vi "tm3samp_sequence_wDSP.vi"() -> ()   [LabVIEW 2011]
panel:
  in  "SC Enable":bool
  in  "BG Enable":bool
  in  "Frame Averaging":i32(ring)=1 items=["1 Frame"=1, "2 Frames"=2, "4 Frames"=4]
  in  "Recursive Frames":i32(ring)=1 items=["1 Frame"=1, "2 Frames"=2, "4 Frames"=4, "8 Frames"=8, "16 Frames"=16]
  out "Image":u16[][](graph)
  in  "Quit":bool
  out "Error Out":errorcluster {"code" format="%.0x"}
  # "This is an example how to use the DSP functions.\nNot all camera have the DSP functions. Please\ncheck your camera manual to see your camera's\ncapabilities."
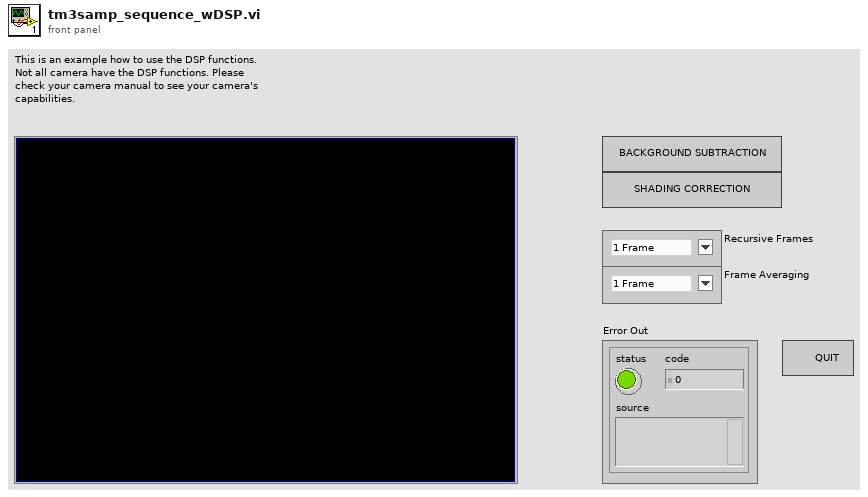
[diagram p1: front panel]
types:
  T1 = cluster{"width":u32, "height":u32, "datatype":u32}
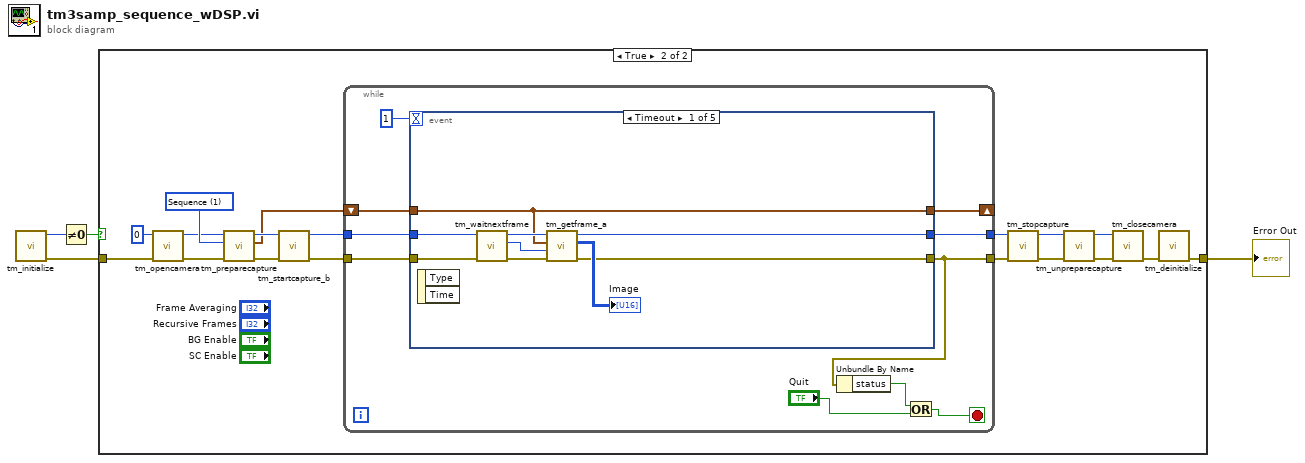
[diagram p0: block diagram]
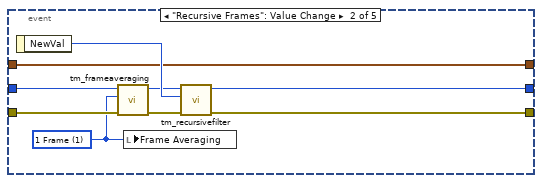
[diagram p3: hidden frame]
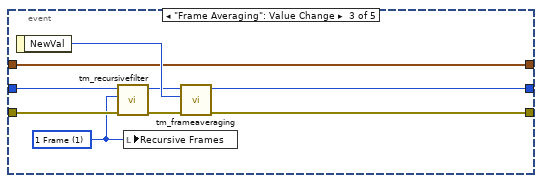
[diagram p4: hidden frame]
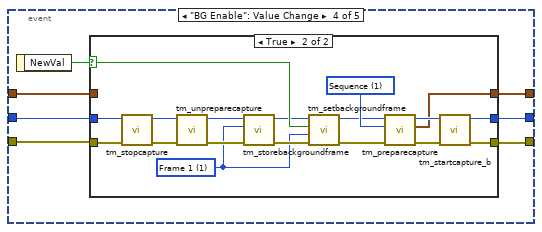
[diagram p5: hidden frame]
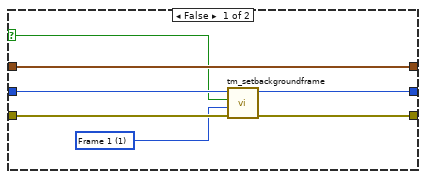
[diagram p6: hidden frame]
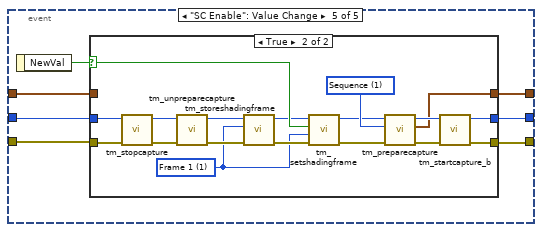
[diagram p7: hidden frame]
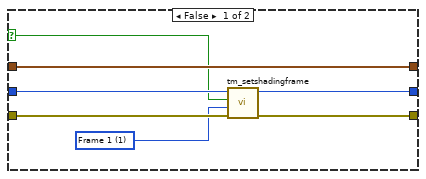
[diagram p8: hidden frame]
diagram:
  n1 = call <userlib>:"tm_initialize.vi"() -> ("error out"=w1:errorcluster, "Number Of Cameras"=w2:u32)  [unwired: 10 in]
  n2 = Not Equal To 0?(x=w2) -> (x != 0?=w4:bool)
  n3 = case shown="True" w4 {
    tunnel: w1 -> [w5 w23]
    tunnel: [w5 w20] -> w3
    frame False {
    }
    frame True {
      w13 = 1 items=["Snap", "Sequence"] ("Capture mode")
      n4 = call <userlib>:"tm_opencamera.vi"("error in (no error)"=w23, "Camera Index"=u32 0) -> ("error out"=w10:errorcluster, "Handle out"=w9:u32)  [unwired: 8 in]
      n5 = call <userlib>:"tm_preparecapture.vi"("error in (no error)"=w10, "Capture mode"=w13, "Handle in"=w9) -> ("error out"=w11:errorcluster, "Buffer"=w6:T1, "Handle out"=w12:u32)  [unwired: 5 in, 1 out]
      n6 = call <userlib>:"tm_startcapture_b.vi"("error in (no error)"=w11, "Handle in"=w12) -> ("error out"=w7:errorcluster, "Handle out"=w8:u32)  [unwired: 8 in]
      n7 = while {
        tunnel: [w31] -> w16
        tunnel: [w26] -> w17
        tunnel: w8 -> [w33]
        tunnel: w7 -> [w32]
        shift-right: [w25] -> _
        shift-left: w6 -> [w30]
        stop <- w24 stop-if-true
        n8 = event shown="[0] Timeout" {
          selector: _ -> [_ _ _ _ _]
          dyn-events: _ -> [_ _ _ _ _]
          timeout: 1 -> [_ _ _ _ _]
          tunnel: w33 -> [w38 w47 w56 w65 w97]
          tunnel: w32 -> [w37 w48 w57 w64 w96]
          tunnel: [w35 w50 w59 w62 w94] -> w31
          tunnel: [w36 w49 w58 w61 w93] -> w26
          tunnel: w30 -> [w34 w43 w52 w66 w98]
          tunnel: [w34 w43 w52 w63 w95] -> w25
          event Timeout {
            n9 = event-data() -> ()  [unwired: 1 in, 2 out]
            n10 = call <userlib>:"tm_waitnextframe.vi"("error in (no error)"=w37, "Handle in"=w38) -> ("error out"=w40:errorcluster, "Frame Index"=w42:i32, "Handle out"=w39:u32)  [unwired: 6 in, 1 out]
            n11 = call <userlib>:"tm_getframe_a.vi"("error in (no error)"=w40, "Frame Index"=w42, "Buffer"=w34, "Handle in"=w39) -> ("error out"=w36:errorcluster, "Data 16"=→"Image":u16[][], "Handle out"=w35:u32)  [unwired: 3 in, 2 out]
          }
          event "Recursive Frames": Value Change {
            w44 = 1 items=["1 Frame"=1, "2 Frames"=2, "4 Frames"=4, "8 Frames"=8, "16 Frames"=16] ("Frames")
            n12 = event-data() -> ("NewVal"=w51:i32)  [unwired: 1 in]
            n13 = call <userlib>:"tm_frameaveraging.vi"("error in (no error)"=w48, "Frames"=w44, "Handle in"=w47) -> ("error out"=w45:errorcluster, "Handle out"=w46:u32)  [unwired: 7 in]
            n14 = local write "Frame Averaging"(w44) -> ()
            n15 = call <userlib>:"tm_recursivefilter.vi"("error in (no error)"=w45, "Frames"=w51, "Handle in"=w46) -> ("error out"=w49:errorcluster, "Handle out"=w50:u32)  [unwired: 7 in]
          }
          event "Frame Averaging": Value Change {
            w53 = 1 items=["1 Frame"=1, "2 Frames"=2, "4 Frames"=4, "8 Frames"=8, "16 Frames"=16] ("Frames")
            n16 = event-data() -> ("NewVal"=w60:i32)  [unwired: 1 in]
            n17 = call <userlib>:"tm_recursivefilter.vi"("error in (no error)"=w57, "Frames"=w53, "Handle in"=w56) -> ("error out"=w54:errorcluster, "Handle out"=w55:u32)  [unwired: 7 in]
            n18 = local write "Recursive Frames"(w53) -> ()
            n19 = call <userlib>:"tm_frameaveraging.vi"("error in (no error)"=w54, "Frames"=w60, "Handle in"=w55) -> ("error out"=w58:errorcluster, "Handle out"=w59:u32)  [unwired: 7 in]
          }
          event "BG Enable": Value Change {
            n20 = event-data() -> ("NewVal"=w67:bool)  [unwired: 1 in]
            n21 = case shown="True" w67 {
              selector: w67 -> [w68 w86]
              tunnel: w65 -> [w74 w89]
              tunnel: w64 -> [w73 w90]
              tunnel: [w72 w77] -> w62
              tunnel: [w71 w76] -> w61
              tunnel: w66 -> [w70 _]
              tunnel: [w70 w75] -> w63
              frame False {
                w69 = 1 items=["Frame 1"=1, "Frame 2"=2, "Frame 3"=3, "Frame 4"=4] ("Frame")
                n22 = call <userlib>:"tm_setbackgroundframe.vi"("error in (no error)"=w73, "Frame"=w69, "Enable"=w68, "Handle in"=w74) -> ("error out"=w71:errorcluster, "Handle out"=w72:u32)  [unwired: 6 in]
              }
              frame True {
                w80 = 1 items=["Snap", "Sequence"] ("Capture mode")
                w83 = 1 items=["Frame 1"=1, "Frame 2"=2, "Frame 3"=3, "Frame 4"=4] ("Frame")
                n23 = call <userlib>:"tm_stopcapture.vi"("error in (no error)"=w90, "Handle in"=w89) -> ("error out"=w92:errorcluster, "Handle out"=w91:u32)  [unwired: 8 in]
                n24 = call <userlib>:"tm_unpreparecapture.vi"("error in (no error)"=w92, "Handle in"=w91) -> ("error out"=w87:errorcluster, "Handle out"=w88:u32)  [unwired: 8 in]
                n25 = call <userlib>:"tm_storebackgroundframe.vi"("error in (no error)"=w87, "Frame"=w83, "Handle in"=w88) -> ("error out"=w84:errorcluster, "Handle out"=w85:u32)  [unwired: 7 in]
                n26 = call <userlib>:"tm_setbackgroundframe.vi"("error in (no error)"=w84, "Frame"=w83, "Enable"=w86, "Handle in"=w85) -> ("error out"=w79:errorcluster, "Handle out"=w78:u32)  [unwired: 6 in]
                n27 = call <userlib>:"tm_preparecapture.vi"("error in (no error)"=w79, "Capture mode"=w80, "Handle in"=w78) -> ("error out"=w82:errorcluster, "Buffer"=w75:T1, "Handle out"=w81:u32)  [unwired: 5 in, 1 out]
                n28 = call <userlib>:"tm_startcapture_b.vi"("error in (no error)"=w82, "Handle in"=w81) -> ("error out"=w76:errorcluster, "Handle out"=w77:u32)  [unwired: 8 in]
              }
            }
          }
          event "SC Enable": Value Change {
            n29 = event-data() -> ("NewVal"=w99:bool)  [unwired: 1 in]
            n30 = case shown="True" w99 {
              selector: w99 -> [w100 w114]
              tunnel: w97 -> [w106 w121]
              tunnel: w96 -> [w105 w122]
              tunnel: [w104 w117] -> w94
              tunnel: [w103 w116] -> w93
              tunnel: w98 -> [w102 _]
              tunnel: [w102 w115] -> w95
              frame False {
                w101 = 1 items=["Frame 1"=1, "Frame 2"=2, "Frame 3"=3, "Frame 4"=4] ("Frame")
                n31 = call <userlib>:"tm_setshadingframe.vi"("error in (no error)"=w105, "Frame"=w101, "Enable"=w100, "Handle in"=w106) -> ("error out"=w103:errorcluster, "Handle out"=w104:u32)  [unwired: 6 in]
              }
              frame True {
                w118 = 1 items=["Snap", "Sequence"] ("Capture mode")
                w107 = 1 items=["Frame 1"=1, "Frame 2"=2, "Frame 3"=3, "Frame 4"=4] ("Frame")
                n32 = call <userlib>:"tm_stopcapture.vi"("error in (no error)"=w122, "Handle in"=w121) -> ("error out"=w124:errorcluster, "Handle out"=w123:u32)  [unwired: 8 in]
                n33 = call <userlib>:"tm_unpreparecapture.vi"("error in (no error)"=w124, "Handle in"=w123) -> ("error out"=w108:errorcluster, "Handle out"=w111:u32)  [unwired: 8 in]
                n34 = call <userlib>:"tm_storeshadingframe.vi"("error in (no error)"=w108, "Frame"=w107, "Handle in"=w111) -> ("error out"=w109:errorcluster, "Handle out"=w110:u32)  [unwired: 7 in]
                n35 = call <userlib>:"tm_setshadingframe.vi"("error in (no error)"=w109, "Frame"=w107, "Enable"=w114, "Handle in"=w110) -> ("error out"=w112:errorcluster, "Handle out"=w113:u32)  [unwired: 6 in]
                n36 = call <userlib>:"tm_preparecapture.vi"("error in (no error)"=w112, "Capture mode"=w118, "Handle in"=w113) -> ("error out"=w120:errorcluster, "Buffer"=w115:T1, "Handle out"=w119:u32)  [unwired: 5 in, 1 out]
                n37 = call <userlib>:"tm_startcapture_b.vi"("error in (no error)"=w120, "Handle in"=w119) -> ("error out"=w116:errorcluster, "Handle out"=w117:u32)  [unwired: 8 in]
              }
            }
          }
        }
        n38 = Unbundle By Name(w26) -> ("status"=w29:bool)
        n39 = Or(x=w29, y="Quit") -> (x .or. y?=w24:bool)
      }
      n40 = call <userlib>:"tm_stopcapture.vi"("error in (no error)"=w17, "Handle in"=w16) -> ("error out"=w14:errorcluster, "Handle out"=w15:u32)  [unwired: 8 in]
      n41 = call <userlib>:"tm_unpreparecapture.vi"("error in (no error)"=w14, "Handle in"=w15) -> ("error out"=w19:errorcluster, "Handle out"=w18:u32)  [unwired: 8 in]
      n42 = call <userlib>:"tm_closecamera.vi"("error in (no error)"=w19, "Handle in"=w18) -> ("error out"=w21:errorcluster)  [unwired: 9 in]
      n43 = call <userlib>:"tm_deinitialize.vi"("error in (no error)"=w21) -> ("error out"=w20:errorcluster)  [unwired: 10 in]
    }
  }
  "Error Out" <- w3
